vi "GeraSinalRuido.vi"(0 "params":variant, 2 "Tx Aquisicao":dbl, 4 "estadoIn":variant) -> (15 "sinal":waveform(dbl), 18 "estadoOut":variant)   [LabVIEW 2017]
uses:
  Typedefs/Tipo_ParamsRuido.ctl
  <vilib>/measure/macond.llb/IIR Filter for 1 Chan.vi
  <vilib>/Analysis/NI_AALBase.lvlib
  <vilib>/measure/NI_MAPro.lvlib
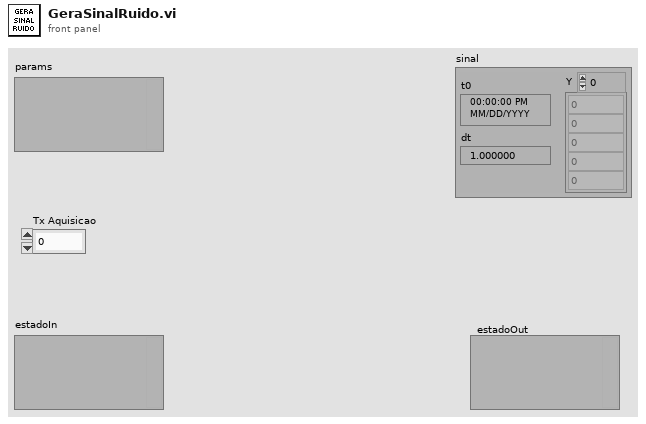
[diagram p1: front panel]
types:
  T1 = cluster{"Topology":enum16{"Off", "Butterworth", "Chebyshev", "Inverse Chebyshev", "Elliptic", "Bessel"}, "Type":enum16{"Lowpass", "Highpass", "Bandpass", "Bandstop"}, "Order":i32, "Lower Fc":dbl, "Upper Fc":dbl, "PB Ripple":dbl, "SB Attenuation":dbl}
  T2 = typedef "Tipo_ParamsRuido.ctl" = cluster{"Amplitude":dbl, "Banda: ":bool, "Freq. Inferior":dbl, "Freq. Superior":dbl}
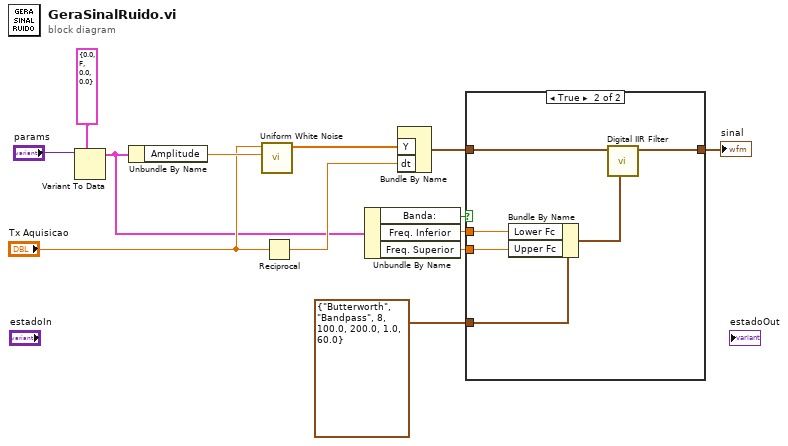
[diagram p0: block diagram]
diagram:
  n1 = Variant To Data(type=T2 {"Amplitude"=0.0, "Banda: "=FALSE, "Freq. Inferior"=0.0, "Freq. Superior"=0.0} ("Tipo_ParamRuido"), Variant="params") -> (data=w7:T2)  [unwired: 1 in, 1 out]
  n2 = Unbundle By Name(w7) -> ("Amplitude"=w11:dbl)
  n3 = call <vilib>:"Uniform White Noise.vi"("amplitude"=w11, "samples"="Tx Aquisicao") -> ("uniform white noise"=w10:dbl[])  [unwired: 8 in, 1 out]
  n4 = Reciprocal(x="Tx Aquisicao") -> (1/x=w8:dbl)
  n5 = Unbundle By Name(w7) -> ("Banda:"=w6:bool, "Freq. Inferior"=w2:dbl, "Freq. Superior"=w1:dbl)
  n6 = Bundle By Name("Y"=w10, "dt"=w8) -> (w5:waveform(dbl))  [unwired: 1 in]
  n7 = case shown="True" w6 {
    tunnel: w5 -> [w14 w20]
    tunnel: [w14 w19] -> w4
    tunnel: T1 {"Topology"=enum."Butterworth", "Type"=enum."Bandpass", "Order"=8, "Lower Fc"=100.0, "Upper Fc"=200.0, "PB Ripple"=1.0, "SB Attenuation"=60.0} ("IIR filter specifications") -> [_ w18]
    tunnel: w2 -> [_ w17]
    tunnel: w1 -> [_ w16]
    frame False {
    }
    frame True {
      n8 = Bundle By Name(cluster=w18, "Lower Fc"=w17, "Upper Fc"=w16) -> (w15:T1)
      n9 = call-poly <vilib>:"Digital IIR Filter.vi"("IIR filter specifications"=w15, "signal in"=w20) -> ("signal out"=w19:waveform(dbl))  [unwired: 7 in, 2 out]
    }
  }
  "sinal" <- w4
